vi "Set Parent Class.vi"(7 "AppInst":refnum<vi>, 8 "error in (no error)":errorcluster, 9 "Parent Class Path":path, 10 "New Class Path":path) -> (0 "error out":errorcluster)   [LabVIEW 2020, in "Message Maker.lvlib"]
uses:
  Message Maker.lvlib
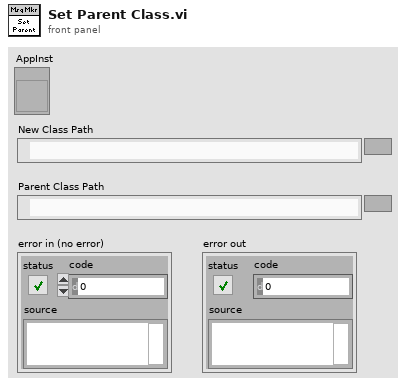
[diagram p1: front panel]
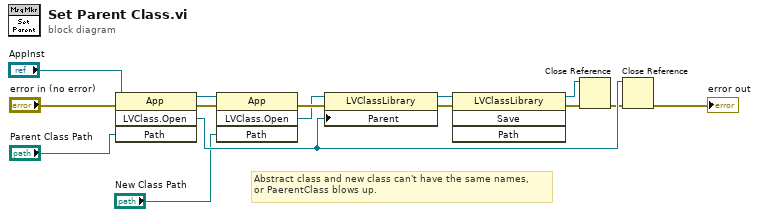
[diagram p0: block diagram]
diagram:
  # "Abstract class and new class can't have the same names,\nor PaerentClass blows up."
  n1 = invoke class="App" method="LVClass.Open"(reference="AppInst", error in="error in (no error)", "Path"="Parent Class Path") -> (reference out=w5:refnum<vi>, error out=w6:errorcluster, "LVClass.Open"=w10:refnum<vi>)  [unwired: 1 in, 1 out]
  n2 = invoke class="App" method="LVClass.Open"(reference=w5, error in=w6, "Path"="New Class Path") -> (error out=w8:errorcluster, "LVClass.Open"=w4:refnum<vi>)  [unwired: 1 in, 2 out]
  n3 = property class="LVClassLibrary"(reference=w4, error in=w8, "Parent"=w10) -> (reference out=w11:refnum<vi>, error out=w12:errorcluster)
  n4 = invoke class="LVClassLibrary" method="Save"(reference=w11, error in=w12) -> (reference out=w14:refnum<vi>, error out=w13:errorcluster)  [unwired: 2 in, 2 out]
  n5 = Close Reference(reference=w14, error in (no error)=w13) -> (error out=w9:errorcluster)
  n6 = Close Reference(reference=w10, error in (no error)=w9) -> (error out=→"error out":errorcluster)
